vi "_io_query_with_OPC_synchro.vi"(1 "Trim Response End":bool=TRUE, 4 "Send *ESR? at the end (T)":bool=TRUE, 5 "Attribute":T1={"Identifier"="", "Descriptive Name"="", "Data Type"=enum."Integer 32", "Command"="", "Access"=enum."Read/Write", "Range Table"="", "Read Callback"="", "Write Callback"="", "Supported Models"="", "Instrument Options"="", "Index"=0, "OPC Wait"=FALSE, "No Status Check"=FALSE, "Cache Only"=FALSE}, 6 "Simulation read buffer (\"Simulation\")":string="Simulation", 7 "Timeout in (0 = OPC timeout)":i32, 8 "error in":errorcluster caption="error in (no error)", 9 "Max segment read bytes count (65536)":u32=65536, 10 "Query":string, 11 "VISA resource name":refnum<visa-resource-name>) -> (0 "error out":errorcluster, 2 "Response":string, 3 "VISA resource name out":refnum<visa-resource-name>)   [LabVIEW 2022 SP3, in "hmp4000_rsidr_core.lvlib"]
uses:
  hmp4000_rsidr_core.lvlib
  type_Attribute.ctl
  type_Attribute_Data_Type.ctl
  type_ReadWriteAccess.ctl
  type_OPC_Wait_Mode.ctl
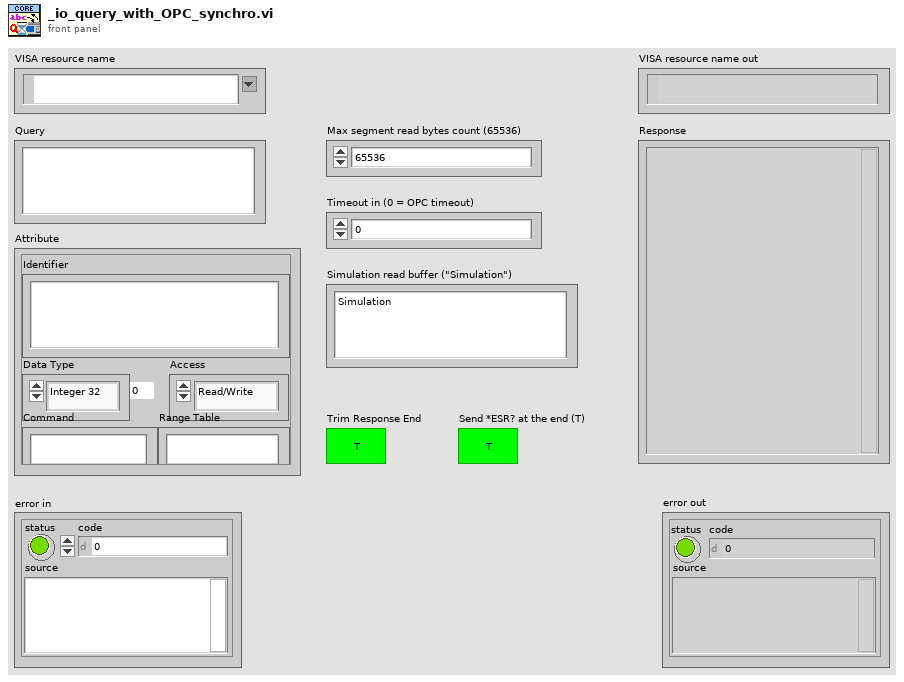
[diagram p1: front panel]
types:
  T1 = typedef "hmp4000_rsidr_core.lvlib/type_Attribute.ctl" = cluster{"Identifier":string, "Descriptive Name":string, "Data Type":T2, "Command":string, "Access":T3, "Range Table":string, "Read Callback":string, "Write Callback":string, "Supported Models":string, "Instrument Options":string, "Index":i32, "OPC Wait":bool, "No Status Check":bool, "Cache Only":bool}
  T2 = typedef "hmp4000_rsidr_core.lvlib/type_Attribute_Data_Type.ctl" = enum16{"Integer 32", "Double", "String", "Boolean", "None", "Integer 64", "RawString"}
  T3 = typedef "hmp4000_rsidr_core.lvlib/type_ReadWriteAccess.ctl" = enum16{"Read Only", "Write Only", "Read/Write"}
  T4 = typedef "hmp4000_rsidr_core.lvlib/type_OPC_Wait_Mode.ctl" = enum16{"STBpolling", "STBpollingSlow", "STBpollingSuperSlow", "ServiceRequest", "OPCquery"}
  T5 = typedef "hmp4000_rsidr_core.lvlib/type_Session_Data.ctl" = cluster{"IDN string":string, "Instrument FW":string, "Instr type":string, "Instr type for err. msg.":string, "Installed Options":string[], "Ignore Error Messages":string, "Logging params":variant, "OPC Timeout":i32, "VISA Timeout":i32, "STB Poll VISA Timeout":i32, "Additional Flags":i32, "Wait Before Read":i32, "Wait Before Write":i32, "Option String Flags":i32, "IO Segment Size":i64, "VISA Access Mode":T6, "Interface Type":T7, "OPC Wait Mode":T4, "Bin Float Number  Format":T8, "Bin Integer Number Format":T9, "Simulate":bool, "VXIcapable":bool, "Duplicate Session":bool, "Add LF to Write":bool, "Logging":bool, "Fast Sweep":bool, "Query Instrument Status":bool, "Check Range":bool, "Check Options":bool}
  T6 = typedef "hmp4000_rsidr_core.lvlib/type_VisaAccessMode.ctl" = u16
  T7 = typedef "hmp4000_rsidr_core.lvlib/type_InterfaceType.ctl" = enum16{"Unknown", "GPIB", "VXI", "GPIB_VXI", "ASRL", "PXI", "TCPIP", "USB", "SOCKET"}
  T8 = typedef "hmp4000_rsidr_core.lvlib/type_Binary_Float_Number_Format.ctl" = enum16{"Float_4_Bytes_Swapped", "Float_4_Bytes", "Double_8_Bytes_Swapped", "Double_8_Bytes"}
  T9 = typedef "hmp4000_rsidr_core.lvlib/type_Binary_Integer_Number_Format.ctl" = enum16{"Int32_4_Bytes_Swapped", "Int32_4 Bytes", "Int16_2_Bytes_Swapped", "Int16_2_Bytes"}
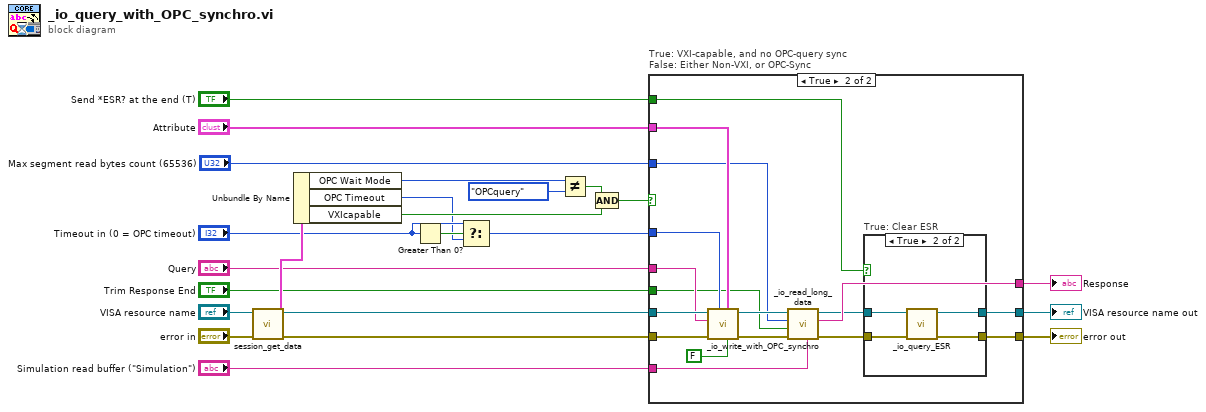
[diagram p0: block diagram]
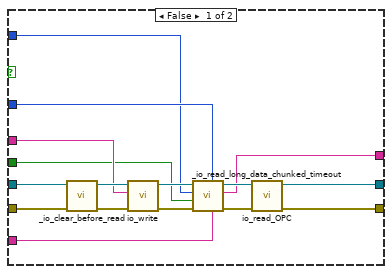
[diagram p2: hidden frame]
diagram:
  n1 = call "session_get_data.vi"("error in"="error in", "VISA resource name"="VISA resource name") -> ("error out"=w15:errorcluster, "Session User Data out"=w21:T5, "VISA resource name out"=w14:refnum<visa-resource-name>)  [unwired: 6 in, 1 out]
  n2 = Unbundle By Name(w21) -> ("OPC Wait Mode"=w20:T4, "OPC Timeout"=w10:i32, "VXIcapable"=w17:bool)
  n3 = Greater Than 0?(x="Timeout in (0 = OPC timeout)") -> (x > 0?=w11:bool)
  n4 = Select(t="Timeout in (0 = OPC timeout)", s=w11, f=w10) -> (s? t:f=w13:i32)
  n5 = Not Equal?(x=w20, y=type_OPC_Wait_Mode."OPCquery") -> (x != y?=w18:bool)
  n6 = Compound Arithmetic op=AND(w18, w17) -> (w16:bool)
  n7 = case "True: VXI-capable, and no OPC-query sync\nFalse: Either Non-VXI, or OPC-Sync" shown="True" w16 {
    tunnel: w15 -> [w39 w56]
    tunnel: w14 -> [w38 w55]
    tunnel: w13 -> [w28 w53]
    tunnel: "Query" -> [w29 w52]
    tunnel: "Attribute" -> [_ w51]
    tunnel: [w31 w43] -> w7
    tunnel: [w30 w42] -> w6
    tunnel: "Max segment read bytes count (65536)" -> [w25 w48]
    tunnel: "Simulation read buffer (\"Simulation\")" -> [w27 w47]
    tunnel: [w26 w46] -> w4
    tunnel: "Send *ESR? at the end (T)" -> [_ w41]
    tunnel: "Trim Response End" -> [w24 w40]
    frame False {
      n8 = call "_io_clear_before_read.vi"("error in"=w39, "VISA resource name"=w38) -> ("error out"=w37:errorcluster, "VISA resource name out"=w36:refnum<visa-resource-name>)  [unwired: 8 in]
      n9 = call "io_write.vi"("error in"=w37, "write buffer"=w29, "VISA resource name"=w36) -> ("error out"=w35:errorcluster, "VISA resource name out"=w34:refnum<visa-resource-name>)  [unwired: 7 in]
      n10 = call "_io_read_long_data_chunked_timeout.vi"("Simulation read buffer (\"Simulation\")"=w27, "Timeout for chunked touts (-1: No chunked touts)"=w28, "error in"=w35, "Trim Response End"=w24, "Max segment read bytes count (65536)"=w25, "VISA resource name"=w34) -> ("error out"=w33:errorcluster, "Read buffer"=w26:string, "VISA resource name out"=w32:refnum<visa-resource-name>)  [unwired: 2 in, 1 out]
      n11 = call "io_read_OPC.vi"("error in"=w33, "VISA resource name"=w32) -> ("error out"=w31:errorcluster, "VISA resource name out"=w30:refnum<visa-resource-name>)  [unwired: 7 in, 1 out]
    }
    frame True {
      n12 = call "_io_write_with_OPC_synchro.vi"("Send *ESR? at the end (T)"=FALSE, "Attribute"=w51, "Timeout in (0 = OPC timeout)"=w53, "error in"=w56, "Write Command"=w52, "VISA resource name"=w55) -> ("error out"=w50:errorcluster, "VISA resource name out"=w49:refnum<visa-resource-name>)  [unwired: 3 in, 1 out]
      n13 = call "_io_read_long_data.vi"("Simulation read buffer (\"Simulation\")"=w47, "error in"=w50, "Trim Response End (T)"=w40, "Max segment read bytes count (65536)"=w48, "VISA resource name"=w49) -> ("error out"=w45:errorcluster, "Read buffer"=w46:string, "VISA resource name out"=w44:refnum<visa-resource-name>)  [unwired: 3 in, 1 out]
      n14 = case "True: Clear ESR" shown="True" w41 {
        tunnel: w45 -> [w58 w62]
        tunnel: w44 -> [w57 w61]
        tunnel: [w58 w60] -> w43
        tunnel: [w57 w59] -> w42
        frame False {
        }
        frame True {
          n15 = call "_io_query_ESR.vi"("error in"=w62, "VISA resource name"=w61) -> ("error out"=w60:errorcluster, "VISA resource name out"=w59:refnum<visa-resource-name>)  [unwired: 7 in, 1 out]
        }
      }
    }
  }
  "VISA resource name out" <- w6
  "error out" <- w7
  "Response" <- w4
